vi "Reset.vi"(11 "handler in":refnum<class "Handler.lvclass">) -> (2 "successful?":bool, 3 "handler out":refnum<class "Handler.lvclass">)   [LabVIEW 2024, in "Logging.lvlib" / "Handler.lvclass"]
uses:
  Handler.lvclass
  Handler.lvclass/Handler.ctl
panel:
  # "Connector Pane"
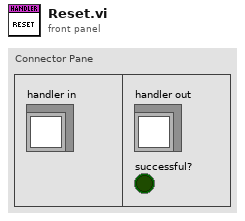
[diagram p1: front panel]
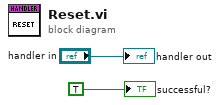
[diagram p0: block diagram]
diagram:
  "handler out" <- "handler in"
  "successful?" <- TRUE ("successful?")
